vi "onCreate.vi"(8 "error in (no error)":errorcluster, 11 "MQTT_Base in":refnum<class "MQTT_Base.lvclass">) -> (0 "error out":errorcluster, 3 "MQTT_Base out":refnum<class "MQTT_Base.lvclass">)   [LabVIEW 2013, in "MQTT Base.lvlib" / "MQTT_Base.lvclass"]
uses:
  MQTT_Base.lvclass
  Request -- cluster.ctl
  <vilib>/LabVIEW Open Source Project/MQTT Control Packets/Control Packets/ControlPacket/ControlPacket.lvclass
  Response -- cluster.ctl
  Subscription/Subscription.lvclass
  <vilib>/LabVIEW Open Source Project/MQTT Control Packets/Control Packets/PUBLISH/PUBLISH.lvclass
  Public Events -- cluster.ctl
  MQTT_Base.lvclass/MQTT_Base.ctl
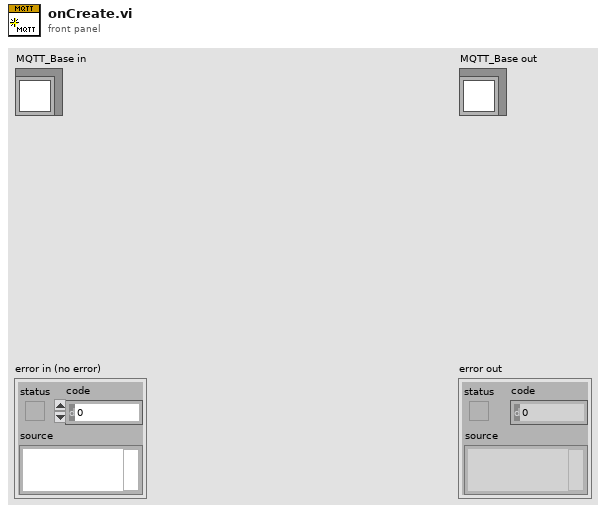
[diagram p1: front panel]
types:
  T1 = typedef "MQTT Base.lvlib/MQTT_Base.lvclass/Public Events -- cluster.ctl" = cluster{"Stop Event":refnum<user-event>, "Error Event":refnum<user-event>, "Inbound Message":refnum<user-event>}
  T2 = typedef "MQTT Base.lvlib/MQTT_Base.lvclass/Request -- cluster.ctl" = cluster{"Packet":refnum<class "ControlPacket.lvclass">, "SessionMailbox":refnum<queue>}
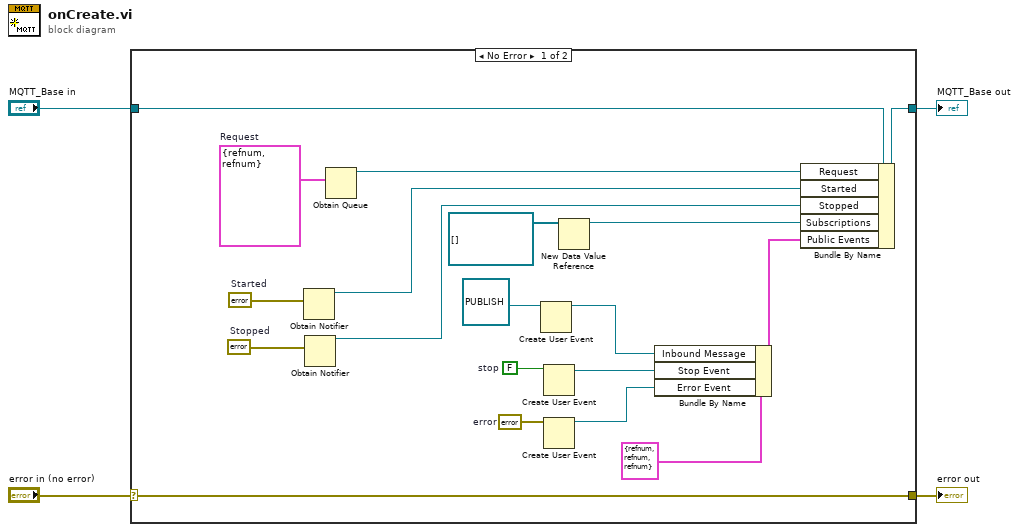
[diagram p0: block diagram]
diagram:
  n1 = case shown="No Error" "error in (no error)" {
    selector: "error in (no error)" -> [w23 w25]
    tunnel: [w23 w25] -> w3
    tunnel: [w17 w24] -> w1
    tunnel: "MQTT_Base in" -> [w18 w24]
    frame No Error {
      w7 = errorcluster {"status"=FALSE, "code"=0, "source"=""}  # error
      w8 = FALSE  # stop
      w12 = errorcluster {"status"=FALSE, "code"=0, "source"=""}  # Stopped
      w13 = errorcluster {"status"=FALSE, "code"=0, "source"=""}  # Started
      w22 = T2 {"Packet"=refnum, "SessionMailbox"=refnum}  # Request
      n2 = Obtain Notifier(notification data type=w13) -> (notifier out=w20:refnum<notifier>)  [unwired: 3 in, 2 out]
      n3 = Obtain Notifier(notification data type=w12) -> (notifier out=w19:refnum<notifier>)  [unwired: 3 in, 2 out]
      n4 = Obtain Queue(element data type=w22) -> (queue out=w21:refnum<queue>)  [unwired: 4 in, 2 out]
      n5 = Create User Event(user event datatype=refnum<class "PUBLISH.lvclass"> refnum ("PUBLISH.lvclass")) -> (user event=w5:refnum<user-event>)  [unwired: 1 in, 1 out]
      n6 = Create User Event(user event datatype=w8) -> (user event=w10:refnum<user-event>)  [unwired: 1 in, 1 out]
      n7 = Create User Event(user event datatype=w7) -> (user event=w9:refnum<user-event>)  [unwired: 1 in, 1 out]
      n8 = New Data Value Reference(data value=refnum<class "Subscription.lvclass">[] []) -> (data value reference=w15:refnum<data-value>)  [unwired: 1 in, 1 out]
      n9 = Bundle By Name(cluster=T1 {"Stop Event"=refnum, "Error Event"=refnum, "Inbound Message"=refnum} ("Public Events"), "Inbound Message"=w5, "Stop Event"=w10, "Error Event"=w9) -> (w6:T1)
      n10 = Bundle By Name(cluster=w18, "Request"=w21, "Started"=w20, "Stopped"=w19, "Subscriptions"=w15, "Public Events"=w6) -> (w17:refnum<class "MQTT_Base.lvclass">)
    }
    frame Error {
    }
  }
  "error out" <- w3
  "MQTT_Base out" <- w1
